vi "Main.vi"(8 "error in (no error)":errorcluster, 10 "Temperature_Notifier":refnum<notifier>, 11 "Message Queues":T1) -> (0 "error out":errorcluster)   [LabVIEW 2019, in "Alarm_Manager.lvlib"]
uses:
  Alarm_Manager.lvlib
  Framework/Message Queue/All Message Queues.ctl
  Framework/Message Queue/Message Cluster.ctl
  Alarm_Data.ctl
  Message_Handler/typedef/Alarm_Panel.ctl
  Channel_Temperature_Threshold.ctl
  Open_Circuit.ctl
  <vilib>/Utility/sysdir.llb/System Directory Type.ctl
  Framework/Message Queue/Enqueue Message (Single).vi
  Framework/Message Queue/Message Queue.lvlib
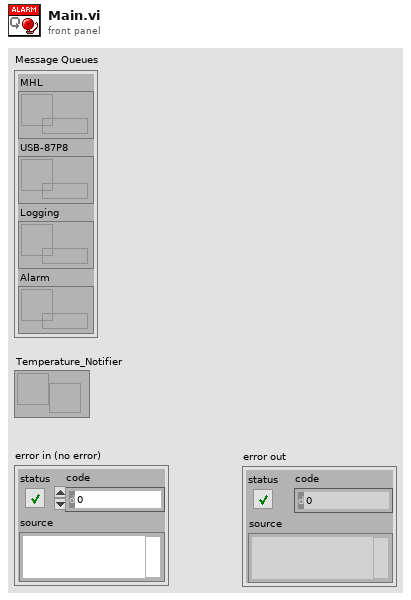
[diagram p1: front panel]
types:
  T1 = typedef "Message Queue.lvlib/All Message Queues.ctl" = cluster{"MHL":refnum<queue>, "USB-87P8":refnum<queue>, "Logging":refnum<queue>, "Alarm":refnum<queue>}
  T2 = typedef "Alarm_Data.ctl" = cluster{"Alarm Panel":T3, "Alarm_State":bool, "Config_Path":path, "Open Circuit":T5}
  T3 = typedef "Alarm_Panel.ctl" = cluster{"Channel (0 - 7)":cluster{"Channel Temperature Thresholds":T4, "Channel Temperature Thresholds 2":T4, "Channel Temperature Thresholds 3":T4, "Channel Temperature Thresholds 4":T4, "Channel Temperature Thresholds 5":T4, "Channel Temperature Thresholds 6":T4, "Channel Temperature Thresholds 7":T4, "Channel Temperature Thresholds 8":T4}, "Channel (8 - 15)":cluster{"Channel Temperature Thresholds":T4, "Channel Temperature Thresholds 2":T4, "Channel Temperature Thresholds 3":T4, "Channel Temperature Thresholds 4":T4, "Channel Temperature Thresholds 5":T4, "Channel Temperature Thresholds 6":T4, "Channel Temperature Thresholds 7":T4, "Channel Temperature Thresholds 8":T4}, "Channel (16 - 23)":cluster{"Channel Temperature Thresholds":T4, "Channel Temperature Thresholds 2":T4, "Channel Temperature Thresholds 3":T4, "Channel Temperature Thresholds 4":T4, "Channel Temperature Thresholds 5":T4, "Channel Temperature Thresholds 6":T4, "Channel Temperature Thresholds 7":T4, "Channel Temperature Thresholds 8":T4}, "Channel (24 - 31)":cluster{"Channel Temperature Thresholds":T4, "Channel Temperature Thresholds 2":T4, "Channel Temperature Thresholds 3":T4, "Channel Temperature Thresholds 4":T4, "Channel Temperature Thresholds 5":T4, "Channel Temperature Thresholds 6":T4, "Channel Temperature Thresholds 7":T4, "Channel Temperature Thresholds 8":T4}}
  T4 = typedef "Channel_Temperature_Threshold.ctl" = cluster{"Min":i32, "Max":i32, "Alarm":i32, "Status":u32}
  T5 = typedef "Open_Circuit.ctl" = cluster{"Temperature":i32, "Thermocouple":i32, "IsOpenCircuit":bool}
  T6 = typedef "System Directory Type.ctl" = i32
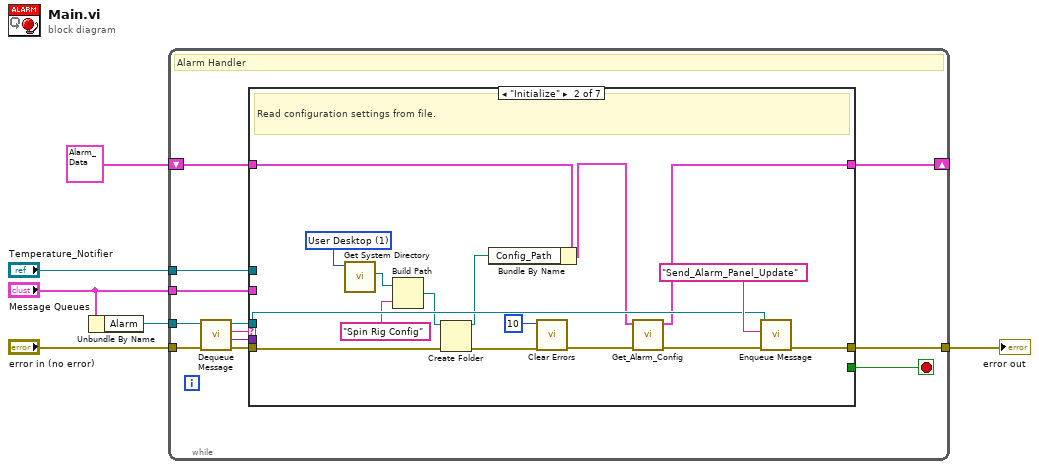
[diagram p0: block diagram]
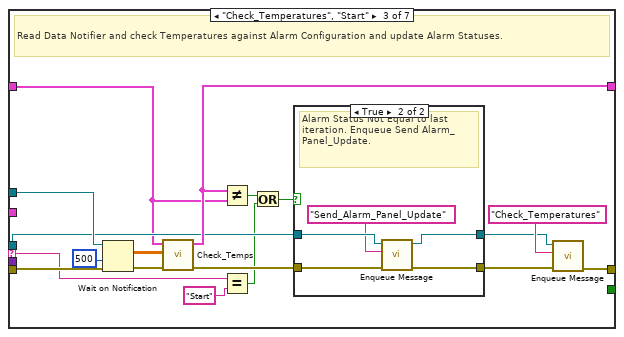
[diagram p3: hidden frame]
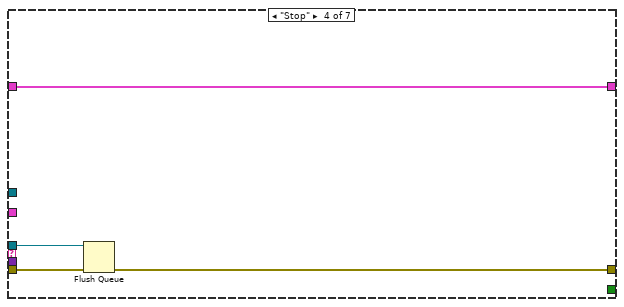
[diagram p5: hidden frame]
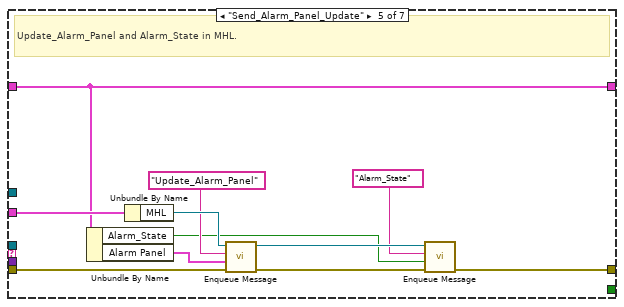
[diagram p6: hidden frame]
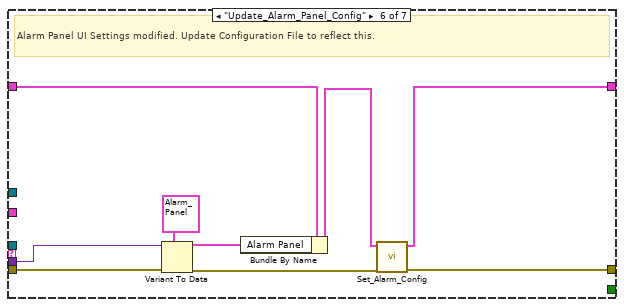
[diagram p7: hidden frame]
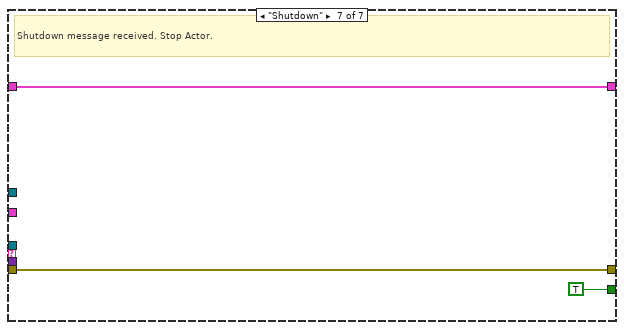
[diagram p8: hidden frame]
diagram:
  n1 = Unbundle By Name("Message Queues") -> ("Alarm"=w3:refnum<queue>)
  n2 = while {
    tunnel: "error in (no error)" -> [w18]
    tunnel: "Message Queues" -> [w13]
    tunnel: w3 -> [w17]
    tunnel: [w12] -> w5
    shift-right: [w9] -> _
    shift-left: T2 {"Alarm Panel"={"Channel (0 - 7)"={"Channel Temperature Thresholds"={"Min"=0, "Max"=0, "Alarm"=0, "Status"=0}, "Channel Temperature Thresholds 2"={"Min"=0, "Max"=0, "Alarm"=0, "Status"=0}, "Channel Temperature Thresholds 3"={"Min"=0, "Max"=0, "Alarm"=0, "Status"=0}, "Channel Temperature Thresholds 4"={"Min"=0, "Max"=0, "Alarm"=0, "Status"=0}, "Channel Temperature Thresholds 5"={"Min"=0, "Max"=0, "Alarm"=0, "Status"=0}, "Channel Temperature Thresholds 6"={"Min"=0, "Max"=0, "Alarm"=0, "Status"=0}, "Channel Temperature Thresholds 7"={"Min"=0, "Max"=0, "Alarm"=0, "Status"=0}, "Channel Temperature Thresholds 8"={"Min"=0, "Max"=0, "Alarm"=0, "Status"=0}}, "Channel (8 - 15)"={"Channel Temperature Thresholds"={"Min"=0, "Max"=0, "Alarm"=0, "Status"=0}, "Channel Temperature Thresholds 2"={"Min"=0, "Max"=0, "Alarm"=0, "Status"=0}, "Channel Temperature Thresholds 3"={"Min"=0, "Max"=0, "Alarm"=0, "Status"=0}, "Channel Temperature Thresholds 4"={"Min"=0, "Max"=0, "Alarm"=0, "Status"=0}, "Channel Temperature Thresholds 5"={"Min"=0, "Max"=0, "Alarm"=0, "Status"=0}, "Channel Temperature Thresholds 6"={"Min"=0, "Max"=0, "Alarm"=0, "Status"=0}, "Channel Temperature Thresholds 7"={"Min"=0, "Max"=0, "Alarm"=0, "Status"=0}, "Channel Temperature Thresholds 8"={"Min"=0, "Max"=0, "Alarm"=0, "Status"=0}}, "Channel (16 - 23)"={"Channel Temperature Thresholds"={"Min"=0, "Max"=0, "Alarm"=0, "Status"=0}, "Channel Temperature Thresholds 2"={"Min"=0, "Max"=0, "Alarm"=0, "Status"=0}, "Channel Temperature Thresholds 3"={"Min"=0, "Max"=0, "Alarm"=0, "Status"=0}, "Channel Temperature Thresholds 4"={"Min"=0, "Max"=0, "Alarm"=0, "Status"=0}, "Channel Temperature Thresholds 5"={"Min"=0, "Max"=0, "Alarm"=0, "Status"=0}, "Channel Temperature Thresholds 6"={"Min"=0, "Max"=0, "Alarm"=0, "Status"=0}, "Channel Temperature Thresholds 7"={"Min"=0, "Max"=0, "Alarm"=0, "Status"=0}, "Channel Temperature Thresholds 8"={"Min"=0, "Max"=0, "Alarm"=0, "Status"=0}}, "Channel (24 - 31)"={"Channel Temperature Thresholds"={"Min"=0, "Max"=0, "Alarm"=0, "Status"=0}, "Channel Temperature Thresholds 2"={"Min"=0, "Max"=0, "Alarm"=0, "Status"=0}, "Channel Temperature Thresholds 3"={"Min"=0, "Max"=0, "Alarm"=0, "Status"=0}, "Channel Temperature Thresholds 4"={"Min"=0, "Max"=0, "Alarm"=0, "Status"=0}, "Channel Temperature Thresholds 5"={"Min"=0, "Max"=0, "Alarm"=0, "Status"=0}, "Channel Temperature Thresholds 6"={"Min"=0, "Max"=0, "Alarm"=0, "Status"=0}, "Channel Temperature Thresholds 7"={"Min"=0, "Max"=0, "Alarm"=0, "Status"=0}, "Channel Temperature Thresholds 8"={"Min"=0, "Max"=0, "Alarm"=0, "Status"=0}}}, "Alarm_State"=FALSE, "Config_Path"=path "", "Open Circuit"={"Temperature"=0, "Thermocouple"=0, "IsOpenCircuit"=FALSE}} -> [w10]
    tunnel: "Temperature_Notifier" -> [w7]
    stop <- w11 stop-if-true
    # "Alarm Handler"
    n3 = call "Dequeue Message.vi"("error in (no error)"=w18, "Message Queue"=w17) -> ("error out"=w14:errorcluster, "Message Data"=w8:variant, "Message"=w15:string, "dup Message Queue"=w16:refnum<queue>)  [unwired: 6 in]
    n4 = case shown="\"Initialize\"" w15 {
      selector: w15 -> [_ _ w41 _ _ _ _]
      tunnel: w16 -> [_ w34 w44 w64 _ _ _]
      tunnel: w14 -> [w20 w27 w53 w65 w76 w83 w88]
      tunnel: w13 -> [_ _ _ _ w75 _ _]
      tunnel: [w20 w36 w51 w63 w69 w77 w88] -> w12
      tunnel: [_ _ _ _ _ _ TRUE] -> w11
      tunnel: w10 -> [w19 w26 w42 w62 w71 w85 w86]
      tunnel: [w19 w32 w47 w62 w71 w78 w86] -> w9
      tunnel: w8 -> [_ _ _ _ _ w79 _]
      tunnel: w7 -> [_ _ w54 _ _ _ _]
      frame Default {
        # "Unknown message received."
      }
      frame "Initialize" {
        w28 = T6 1 items=["User Home"=0, "User Desktop"=1, "User Documents"=2, "User Application Data"=3, "User Preferences"=4, "User Temporary"=5, "Public Documents"=6, "Public Application Data"=7, "Public Preferences"=8, "Public Cache"=13, "System Core Libraries"=9, "System Installed Libraries"=10, "Application Files"=11, "Boot Volume Root"=12] ("system directory type")
        # "Read configuration settings from file."
        n5 = call <vilib>:"Get System Directory.vi"("system directory type"=w28) -> ("system directory"=w29:path)  [unwired: 10 in]
        n6 = Build Path(base path=w29, name or relative path="Spin Rig Config") -> (appended path=w30:path)
        n7 = Create Folder(path (use dialog)=w30, error in=w27) -> (created path=w25:path, error out=w22:errorcluster)  [unwired: 1 in, 1 out]
        n8 = Bundle By Name(cluster=w26, "Config_Path"=w25) -> (w24:T2)
        n9 = call <vilib>:"Clear Errors.vi"("error in (no error)"=w22, "specific error code to clear (0: all)"=10) -> ("error out"=w23:errorcluster)  [unwired: 4 in, 1 out]
        n10 = call "Get_Alarm_Config.vi"("error in (no error)"=w23, "Alarm_Data In"=w24) -> ("error out"=w33:errorcluster, "Alarm_Data Out"=w32:T2)  [unwired: 8 in]
        n11 = call-poly "Enqueue Message.vi"("error in (no error)"=w33, "Message"="Send_Alarm_Panel_Update", "Message Queue"=w34) -> ("error out"=w36:errorcluster)  [unwired: 7 in, 1 out]
      }
      frame "Check_Temperatures", "Start" {
        # "Read Data Notifier and check Temperatures against Alarm Configuration and update Alarm Statuses."
        n12 = Wait on Notification(notifier=w54, timeout in ms (-1)=500, error in (no error)=w53) -> (notification=w48:sgl[][], error out=w49:errorcluster)  [unwired: 1 in, 2 out]
        n13 = call "Check_Temps.vi"("error in (no error)"=w49, "Temperatures"=w48, "Alarm_Data In"=w42) -> ("error out"=w46:errorcluster, "Alarm_Data out"=w47:T2)  [unwired: 7 in]
        n14 = Not Equal?(x=w47, y=w42) -> (x != y?=w39:bool)
        n15 = Equal?(x=w41, y="Start") -> (x = y?=w38:bool)
        n16 = Or(x=w39, y=w38) -> (x .or. y?=w37:bool)
        n17 = case shown="True" w37 {
          tunnel: w46 -> [w55 w61]
          tunnel: [w55 w60] -> w45
          tunnel: w44 -> [w56 w59]
          tunnel: [w56 w58] -> w43
          frame False {
            # "Alarm Statuses have not changed."
          }
          frame True {
            # "Alarm Status Not Equal to last iteration. Enqueue Send Alarm_Panel_Update."
            n18 = call-poly "Enqueue Message.vi"("error in (no error)"=w61, "Message"="Send_Alarm_Panel_Update", "Message Queue"=w59) -> ("error out"=w60:errorcluster, "dup Message Queue"=w58:refnum<queue>)  [unwired: 7 in]
          }
        }
        n19 = call-poly "Enqueue Message.vi"("error in (no error)"=w45, "Message"="Check_Temperatures", "Message Queue"=w43) -> ("error out"=w51:errorcluster)  [unwired: 7 in, 1 out]
      }
      frame "Stop" {
        n20 = Flush Queue(queue=w64, error in (no error)=w65) -> (error out=w63:errorcluster)  [unwired: 2 out]
      }
      frame "Send_Alarm_Panel_Update" {
        # "Update_Alarm_Panel and Alarm_State in MHL."
        n21 = Unbundle By Name(w71) -> ("Alarm_State"=w66:bool, "Alarm Panel"=w72:T3)
        n22 = Unbundle By Name(w75) -> ("MHL"=w74:refnum<queue>)
        n23 = call-poly "Enqueue Message.vi"("error in (no error)"=w76, "Message Data"=w72, "Message"="Update_Alarm_Panel", "Message Queue"=w74) -> ("error out"=w70:errorcluster, "dup Message Queue"=w68:refnum<queue>)  [unwired: 6 in]
        n24 = call-poly "Enqueue Message.vi"("error in (no error)"=w70, "Message Data"=w66, "Message"="Alarm_State", "Message Queue"=w68) -> ("error out"=w69:errorcluster)  [unwired: 6 in, 1 out]
      }
      frame "Update_Alarm_Panel_Config" {
        # "Alarm Panel UI Settings modified. Update Configuration File to reflect this."
        n25 = Variant To Data(error in=w83, type=T3 {"Channel (0 - 7)"={"Channel Temperature Thresholds"={"Min"=0, "Max"=0, "Alarm"=0, "Status"=0}, "Channel Temperature Thresholds 2"={"Min"=0, "Max"=0, "Alarm"=0, "Status"=0}, "Channel Temperature Thresholds 3"={"Min"=0, "Max"=0, "Alarm"=0, "Status"=0}, "Channel Temperature Thresholds 4"={"Min"=0, "Max"=0, "Alarm"=0, "Status"=0}, "Channel Temperature Thresholds 5"={"Min"=0, "Max"=0, "Alarm"=0, "Status"=0}, "Channel Temperature Thresholds 6"={"Min"=0, "Max"=0, "Alarm"=0, "Status"=0}, "Channel Temperature Thresholds 7"={"Min"=0, "Max"=0, "Alarm"=0, "Status"=0}, "Channel Temperature Thresholds 8"={"Min"=0, "Max"=0, "Alarm"=0, "Status"=0}}, "Channel (8 - 15)"={"Channel Temperature Thresholds"={"Min"=0, "Max"=0, "Alarm"=0, "Status"=0}, "Channel Temperature Thresholds 2"={"Min"=0, "Max"=0, "Alarm"=0, "Status"=0}, "Channel Temperature Thresholds 3"={"Min"=0, "Max"=0, "Alarm"=0, "Status"=0}, "Channel Temperature Thresholds 4"={"Min"=0, "Max"=0, "Alarm"=0, "Status"=0}, "Channel Temperature Thresholds 5"={"Min"=0, "Max"=0, "Alarm"=0, "Status"=0}, "Channel Temperature Thresholds 6"={"Min"=0, "Max"=0, "Alarm"=0, "Status"=0}, "Channel Temperature Thresholds 7"={"Min"=0, "Max"=0, "Alarm"=0, "Status"=0}, "Channel Temperature Thresholds 8"={"Min"=0, "Max"=0, "Alarm"=0, "Status"=0}}, "Channel (16 - 23)"={"Channel Temperature Thresholds"={"Min"=0, "Max"=0, "Alarm"=0, "Status"=0}, "Channel Temperature Thresholds 2"={"Min"=0, "Max"=0, "Alarm"=0, "Status"=0}, "Channel Temperature Thresholds 3"={"Min"=0, "Max"=0, "Alarm"=0, "Status"=0}, "Channel Temperature Thresholds 4"={"Min"=0, "Max"=0, "Alarm"=0, "Status"=0}, "Channel Temperature Thresholds 5"={"Min"=0, "Max"=0, "Alarm"=0, "Status"=0}, "Channel Temperature Thresholds 6"={"Min"=0, "Max"=0, "Alarm"=0, "Status"=0}, "Channel Temperature Thresholds 7"={"Min"=0, "Max"=0, "Alarm"=0, "Status"=0}, "Channel Temperature Thresholds 8"={"Min"=0, "Max"=0, "Alarm"=0, "Status"=0}}, "Channel (24 - 31)"={"Channel Temperature Thresholds"={"Min"=0, "Max"=0, "Alarm"=0, "Status"=0}, "Channel Temperature Thresholds 2"={"Min"=0, "Max"=0, "Alarm"=0, "Status"=0}, "Channel Temperature Thresholds 3"={"Min"=0, "Max"=0, "Alarm"=0, "Status"=0}, "Channel Temperature Thresholds 4"={"Min"=0, "Max"=0, "Alarm"=0, "Status"=0}, "Channel Temperature Thresholds 5"={"Min"=0, "Max"=0, "Alarm"=0, "Status"=0}, "Channel Temperature Thresholds 6"={"Min"=0, "Max"=0, "Alarm"=0, "Status"=0}, "Channel Temperature Thresholds 7"={"Min"=0, "Max"=0, "Alarm"=0, "Status"=0}, "Channel Temperature Thresholds 8"={"Min"=0, "Max"=0, "Alarm"=0, "Status"=0}}} ("Alarm Panel"), Variant=w79) -> (data=w80:T3, error out=w82:errorcluster)
        n26 = Bundle By Name(cluster=w85, "Alarm Panel"=w80) -> (w84:T2)
        n27 = call "Set_Alarm_Config.vi"("error in (no error)"=w82, "Alarm_Data In"=w84) -> ("error out"=w77:errorcluster, "Alarm_Data Out"=w78:T2)  [unwired: 8 in]
      }
      frame "Shutdown" {
        # "Shutdown message received. Stop Actor."
      }
    }
  }
  "error out" <- w5
